vi "DrawShape.vi"(8 "error in (no error)":errorcluster, 9 "Center Position in":cluster{"x":sgl, "y":sgl}, 10 "Picture in":picture, 11 "CircleShape in":refnum<class "CircleShape.lvclass">) -> (0 "error out":errorcluster, 2 "Picture out":picture, 3 "CircleShape out":refnum<class "CircleShape.lvclass">)   [LabVIEW 2022 SP3, in "CircleShape.lvclass"]
uses:
  CircleShape.lvclass
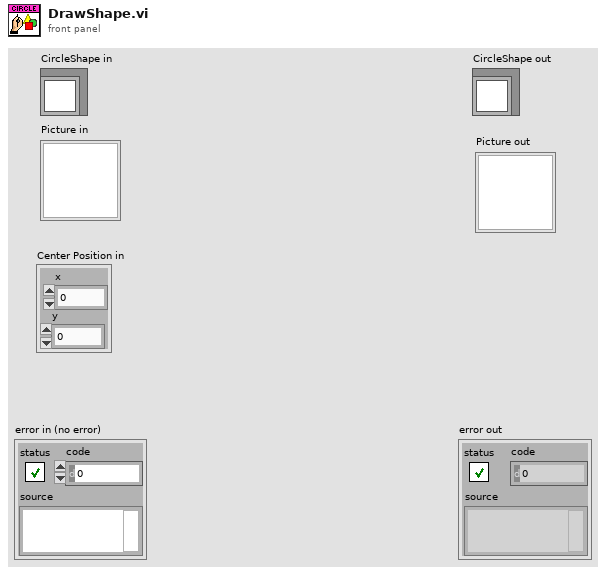
[diagram p1: front panel]
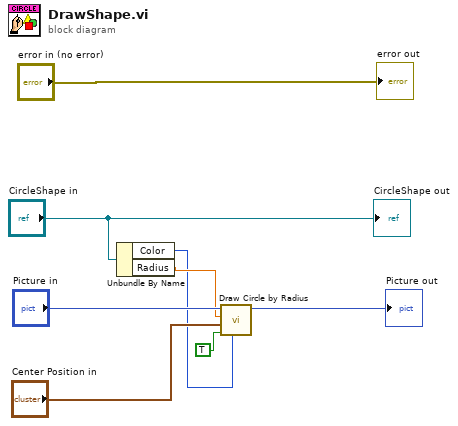
[diagram p0: block diagram]
diagram:
  n1 = Unbundle By Name("CircleShape in") -> ("Color"=w1:u32, "Radius"=w3:dbl)
  n2 = call <vilib>:"Draw Circle by Radius.vi"("color(black)"=w1, "fill?(F)"=TRUE, "pixel center"="Center Position in", "radius"=w3, "picture"="Picture in") -> ("new picture"=→"Picture out":picture)  [unwired: 6 in]
  "error out" <- "error in (no error)"
  "CircleShape out" <- "CircleShape in"
